vi "FindCommonFolder.vi"(10 "Paths":path[](array[path])) -> (2 "common folder":path)   [LabVIEW 2020, in "Caraya.lvlib" / "Test Runner.Folder.lvclass"]
uses:
  Test Runner.Folder.lvclass
  <userlib>/_OpenG.lib/file/file.llb/File Exists - Scalar__ogtk.vi
  <userlib>/_OpenG.lib/file/file.llb/Strip Path - Traditional__ogtk.vi
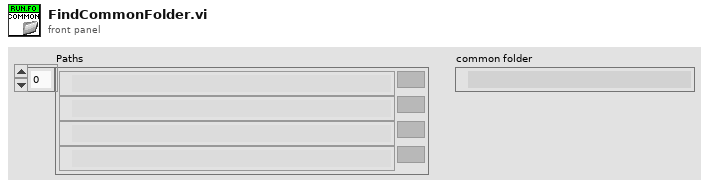
[diagram p1: front panel]
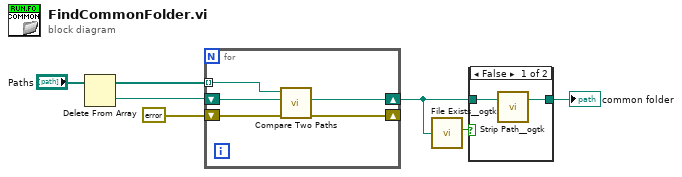
[diagram p0: block diagram]
diagram:
  n1 = Delete From Array(array="Paths") -> (deleted portion=w5:path, array with subset deleted=w2:path[])  [unwired: 2 in]
  n2 = for {
    shift-right: [w10] -> w4
    shift-left: w5 -> [w12]
    tunnel: w2 -> [w11] mode=indexing
    shift-right: [w8] -> _
    shift-left: errorcluster {"status"=FALSE, "code"=0, "source"=""} ("error out") -> [w9]
    n3 = call <vilib>:"Compare Two Paths.vi"("error in (no error)"=w9, "Path 2"=w12, "Path 1"=w11) -> ("error out"=w8:errorcluster, "Common Path"=w10:path)  [unwired: 5 in, 2 out]
  }
  n4 = call-poly <userlib>:"File Exists__ogtk.vi"("file path"=w4) -> ("is directory"=w6:bool)  [unwired: 6 in, 1 out]
  n5 = case shown="False" w6 {
    tunnel: w4 -> [w14 w15]
    tunnel: [w13 w15] -> w3
    frame False {
      n6 = call-poly <userlib>:"Strip Path__ogtk.vi"("path"=w14) -> ("stripped path"=w13:path)  [unwired: 1 out]
    }
    frame True {
    }
  }
  "common folder" <- w3
